vi "SearchCom.vi"(3 "使用注册表？":bool) -> (0 "下拉列表项":cluster{"String":string, "Value":i32}[](array[cluster]))   [LabVIEW 2015]
doc: "利用注册表搜索串口号\n或者使用外部可执行程序搜索串口信息"
uses:
  <vilib>/registry/registry.llb/Registry RtKey.ctl
  <vilib>/registry/registry.llb/Read Registry Value Simple STR.vi
  <vilib>/Utility/config.llb/Read Key (I32).vi
  <vilib>/Utility/config.llb/NI_LVConfig.lvlib
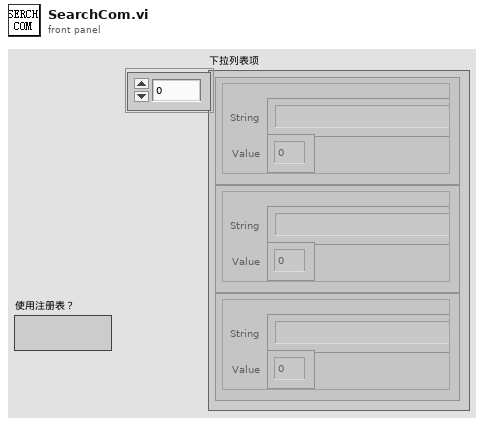
[diagram p1: front panel]
types:
  T1 = typedef "NI_LVConfig.lvlib/Config Data RefNum.ctl" = refnum<k1>
  T2 = typedef "Registry RtKey.ctl" = enum32{"HKEY_CLASSES_ROOT", "HKEY_CURRENT_USER", "HKEY_LOCAL_MACHINE", "HKEY_USERS", "HKEY_PERFORMANCE_DATA", "HKEY_CURRENT_CONFIG", "HKEY_DYN_DATA"}
  T3 = typedef "Registry refnum.ctl" = refnum<k1>
  T4 = cluster{"numValues":i32, "maxValueNameLen":i32, "maxValueDataLen":i32}
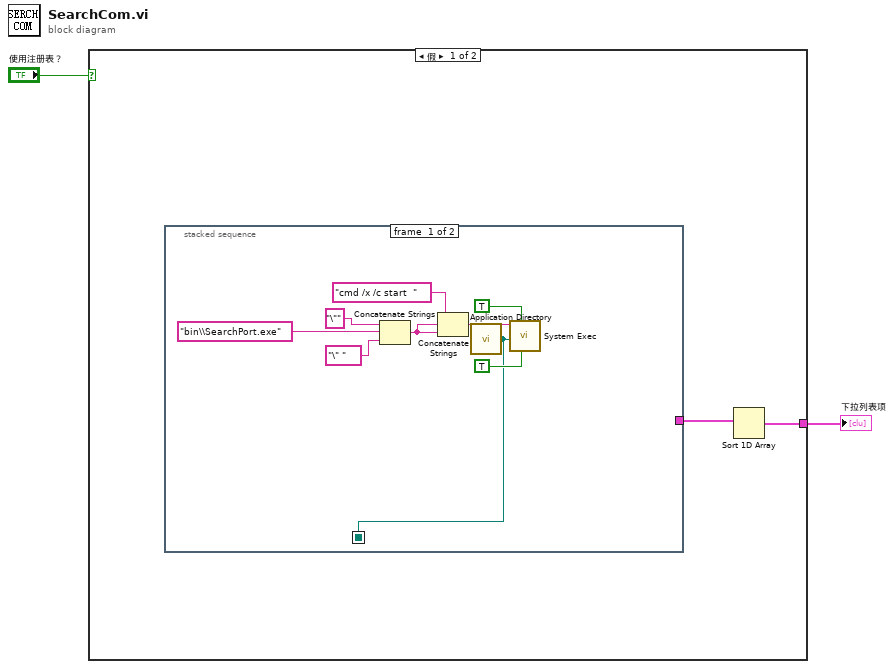
[diagram p0: block diagram]
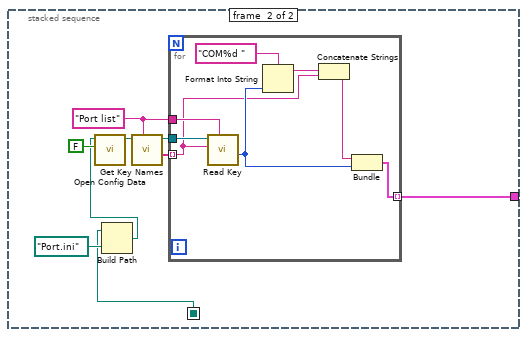
[diagram p2: hidden frame]
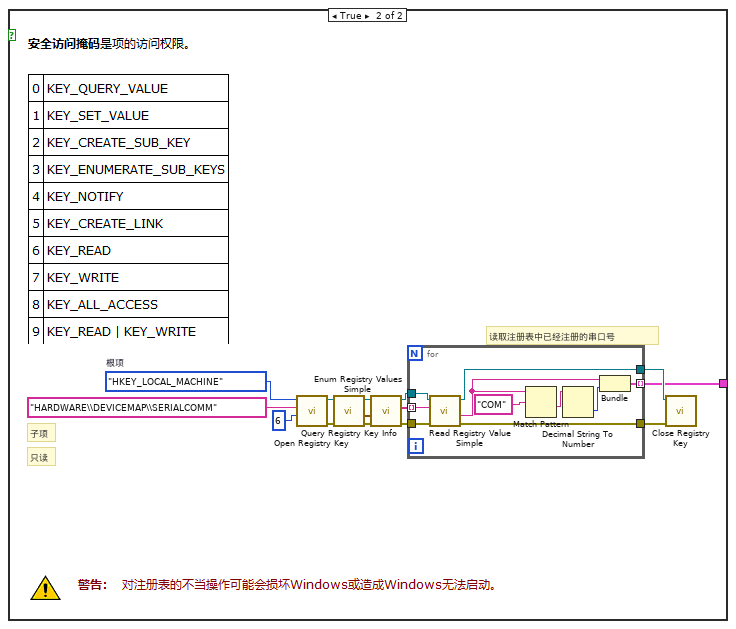
[diagram p3: hidden frame]
diagram:
  n1 = case shown="假" "使用注册表？" {
    tunnel: [w3 w31] -> w1
    frame False {
      n2 = stacked-sequence {
        seq-local: [w5 _] -> [_ w15]
        tunnel: [_ w18] -> w4
        frame #0 {
          n3 = Concatenate Strings("\"" ("Substring"), "bin\\SearchPort.exe", "\" " ("Substring")) -> (w9:string)
          n4 = Concatenate Strings("cmd /x /c start  ", w9, w9) -> (w7:string)
          n5 = call <vilib>:"Application Directory.vi"() -> ("Application Directory"=w5:path)
          n6 = call <vilib>:"System Exec.vi"("run minimized? (F)"=TRUE, "wait until completion? (T)"=TRUE ("Wait until done"), "working directory"=w5, "command line"=w7) -> ()  [unwired: 2 in, 6 out]
        }
        frame #1 {
          w17 = "Port list"
          n7 = Build Path(base path=w15, name or relative path=path "Port.ini" ("default name")) -> (appended path=w14:path)
          n8 = call <vilib>:"Open Config Data.vi"("create file if necessary (T)"=FALSE, "configuration file path"=w14) -> ("refnum"=w21:T1)  [unwired: 7 in, 2 out]
          n9 = call <vilib>:"Get Key Names.vi"("section"=w17, "refnum"=w21) -> ("key names"=w20:string[], "refnum out"=w19:T1)  [unwired: 6 in, 2 out]
          n10 = for {
            tunnel: w20 -> [w24] mode=indexing
            tunnel: w19 -> [w30]
            tunnel: [w29] -> w18 mode=indexing
            tunnel: w17 -> [w28]
            n11 = call-poly <vilib>:"Read Key.vi"("section"=w28, "key"=w24, "refnum"=w30) -> ("value"=w26:i32)  [unwired: 5 in, 3 out]
            n12 = Format Into String(format string="COM%d ", w26) -> (resulting string=w25:string)  [unwired: 2 in, 1 out]
            n13 = Concatenate Strings(w25, w24) -> (w23:string)
            n14 = Bundle(w23, "value"=w26) -> (w29:cluster{string, "value":i32})  [unwired: 1 in]
          }
        }
      }
      n15 = Sort 1D Array(array=w4) -> (sorted array=w3:cluster{string, "value":i32}[])
    }
    frame True {
      w43 = Registry_RtKey."HKEY_LOCAL_MACHINE"  # 根项
      # "只读"
      # "子项"
      # "读取注册表中已经注册的串口号"
      n16 = call <vilib>:"Open Registry Key.vi"("security access mask (KEY_READ | KEY_WRITE)"=u32 6, "subkey"="HARDWARE\\DEVICEMAP\\SERIALCOMM", "root key (HKEY_LOCAL_MACHINE)"=w43) -> ("error out"=w35:errorcluster, "refnum out"=w41:T3)  [unwired: 7 in]
      n17 = call <vilib>:"Query Registry Key Info.vi"("error in (no error)"=w35, "refnum"=w41) -> ("error out"=w34:errorcluster, "value info"=w39:T4, "refnum out"=w40:T3)  [unwired: 5 in, 2 out]
      n18 = call <vilib>:"Enum Registry Values Simple.vi"("error in (no error)"=w34, "value info"=w39, "refnum"=w40) -> ("error out"=w33:errorcluster, "values"=w38:string[], "refnum out"=w37:T3)  [unwired: 3 in, 3 out]
      n19 = for {
        tunnel: w38 -> [w53] mode=indexing
        tunnel: w37 -> [w54]
        tunnel: [w52] -> w36
        tunnel: w33 -> [w51]
        tunnel: [w50] -> w32
        tunnel: [w45] -> w31 mode=indexing
        n20 = call-poly <vilib>:"Read Registry Value Simple.vi"("error in (no error)"=w51, "value"=w53, "refnum"=w54) -> ("error out"=w50:errorcluster, "String/Binary data"=w46:string, "refnum out"=w52:T3)  [unwired: 3 in, 1 out]
        n21 = Match Pattern(string=w46, regular expression="COM") -> (after substring=w48:string)  [unwired: 1 in, 3 out]
        n22 = Decimal String To Number(string=w48) -> (number=w47:i32)  [unwired: 2 in, 1 out]
        n23 = Bundle("String/Binary data"=w46, w47) -> (w45:cluster{"String/Binary data":string, i32})  [unwired: 1 in]
      }
      n24 = call <vilib>:"Close Registry Key.vi"("error in (no error)"=w32, "refnum"=w36) -> ()  [unwired: 5 in, 1 out]
    }
  }
  "下拉列表项" <- w1
